vi "PH_Cont-601k_PSU.Dev Set Flash Interval.vi"(0 "VI in":refnum<vi>, 5 "error in (no error)":errorcluster) -> (14 "VI out":refnum<vi>, 18 "Device Error out":errorcluster, 19 "error out":errorcluster)   [LabVIEW 2014, in "PH_Cont-601k_PSU.lvlib"]
uses:
  PH_Cont-601k_PSU.lvlib
  instr.lib/pu601k/Continuum PU610K.lvlib
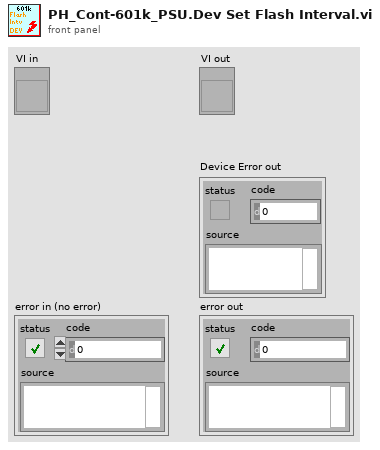
[diagram p1: front panel]
types:
  T1 = typedef "PH_Cont-601k_PSU.lvlib/PH_Cont-601k_PSU.i attribute.ctl" = cluster{"GUI Refs":T2, "Interlock":bool, "Service ID applied Voltage":i32, "Device Settings":cluster{"Configuration":T3, "Flash Interval [s]":dbl, "Mode":T4, "Voltage [V]":u16, "Charge":bool, "VISA resource name":refnum<visa-resource-name>}, "Readyness":T5, "Information":cluster{"VISA resource name":refnum<visa-resource-name>, "Tagname Power On":string, "Interlock":cluster{"Instance":string, "Tagname":string}, "Limits [V]":cluster{"Lower":dbl, "Upper":dbl}, "Tagname PSU On":string}, "R2S":bool, "Charge is allowed":bool}
  T2 = typedef "PH_Cont-601k_PSU.lvlib/PH_Cont-601k_PSU.GUI Refs.ctl" = cluster{"Power On":refnum<vi>, "Hard- and Software":refnum<vi>, "Device Status":refnum<vi>, "Device Error":refnum<vi>, "Configuration":refnum<vi>, "Flash Interval [s]":refnum<vi>, "Interlock":refnum<vi>, "Interlock Indicator":refnum<vi>, "Voltage [V]":refnum<vi>, "Readyness":refnum<vi>, "Mode":refnum<vi>, "Reset Error":refnum<vi>, "Expert working":refnum<vi>, "Charge":refnum<vi>, "PSU On":refnum<vi>}
  T3 = typedef "PH_Cont-601k_PSU.lvlib/PH_Cont-601k_PSU.Configuration.ctl" = u16
  T4 = typedef "PH_Cont-601k_PSU.lvlib/PH_Cont-601k_PSU.Mode.ctl" = enum32{"STOP", "STANDBY", "READY", "EMISSION", "ERROR"}
  T5 = typedef "PH_Cont-601k_PSU.lvlib/PH_Cont-601k_PSU.Readyness.ctl" = cluster{"Program":T6, "Device":T7}
  T6 = typedef "PH_Cont-601k_PSU.lvlib/PH_Cont-601k_PSU.Readyness Program.ctl" = enum32{"OFF", "POWER", "INTERLOCK"}
  T7 = typedef "PH_Cont-601k_PSU.lvlib/PH_Cont-601k_PSU.Readyness Device.ctl" = enum32{"OFF", "CONNECTING", "CONNECTED", "OPERATING", "EOC", "ERROR"}
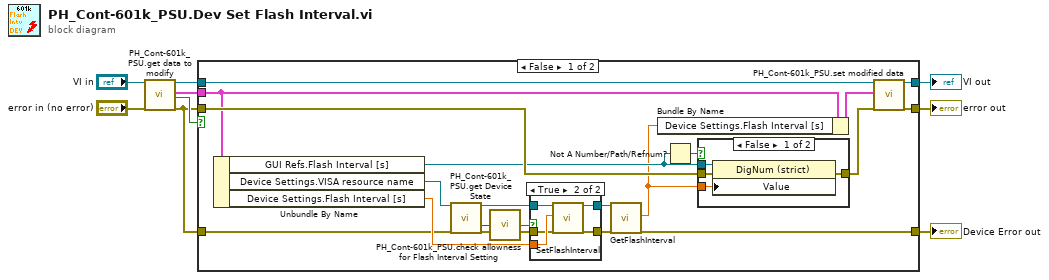
[diagram p0: block diagram]
diagram:
  n1 = call "PH_Cont-601k_PSU.get data to modify.vi"("i ref in"="VI in", "error in (no error)"="error in (no error)") -> ("i ref out"=w5:refnum<vi>, "i attribute"=w8:T1, "timed out"=w2:bool, "error out"=w1:errorcluster)  [unwired: 14 in]
  n2 = case shown="False" w2 {
    tunnel: [w29 w42] -> w9
    tunnel: w8 -> [w16 _]
    tunnel: w1 -> [w26 w42]
    tunnel: w5 -> [w22 w44]
    tunnel: w1 -> [w21 w43]
    tunnel: [w19 w44] -> w4
    tunnel: [w17 w43] -> w3
    frame False {
      n3 = Unbundle By Name(w16) -> ("GUI Refs.Flash Interval [s]"=w20:refnum<vi>, "Device Settings.VISA resource name"=w27:refnum<visa-resource-name>, "Device Settings.Flash Interval [s]"=w28:dbl)
      n4 = call "PH_Cont-601k_PSU.get Device State.vi"("VISA Refnum in"=w27, "Device Error in"=w26) -> ("VISA Refnum out"=w25:refnum<visa-resource-name>, "Device Status: State"=w24:u16, "Device Error out"=w23:errorcluster)  [unwired: 9 in, 6 out]
      n5 = call "PH_Cont-601k_PSU.check allowness for Flash Interval Setting.vi"("Configuration"=w24) -> ("Flash Interval Setting allowed?"=w10:bool)
      n6 = case shown="True" w10 {
        tunnel: w28 -> [_ w36]
        tunnel: w25 -> [w31 w35]
        tunnel: w23 -> [w30 w34]
        tunnel: [w30 w33] -> w15
        tunnel: [w31 w32] -> w14
        frame False {
        }
        frame True {
          n7 = call "SetFlashInterval.vi"("VISA resource name"=w35, "interval (s)"=w36, "error in"=w34) -> ("VISA resource name out"=w32:refnum<visa-resource-name>, "error out"=w33:errorcluster)  [unwired: 15 in]
        }
      }
      n8 = call "GetFlashInterval.vi"("VISA resource name"=w14, "error in"=w15) -> ("interval (s)"=w11:dbl, "error out"=w29:errorcluster)  [unwired: 15 in, 1 out]
      n9 = Bundle By Name(cluster=w16, "Device Settings.Flash Interval [s]"=w11) -> (w12:T1)
      n10 = Not A Number/Path/Refnum?(number/path/refnum=w20) -> (NaN/Path/Refnum?=w13:bool)
      n11 = case shown="False" w13 {
        tunnel: [w40 w41] -> w18
        tunnel: w21 -> [w39 w41]
        tunnel: w20 -> [w38 _]
        tunnel: w11 -> [w37 _]
        frame False {
          n12 = property class="DigNum (strict)"(reference=w38, error in=w39, "Value"=w37) -> (error out=w40:errorcluster)  [unwired: 1 out]
        }
        frame True {
        }
      }
      n13 = call "PH_Cont-601k_PSU.set modified data.vi"("i ref in"=w22, "i attribute"=w12, "error in (no error)"=w18) -> ("i ref out"=w19:refnum<vi>, "error out"=w17:errorcluster)  [unwired: 15 in]
    }
    frame True {
    }
  }
  "error out" <- w3
  "VI out" <- w4
  "Device Error out" <- w9
